vi "RT Driver VI.vi"(7 "Operation":T6, 11 "Device Reference in":T7 format="%.0x") -> (0 "Error Code":i32)   [LabVIEW 2027, in "Embedded Data Logger Engine.lvlib"]
uses:
  Embedded Data Logger Engine.lvlib
  <vilib>/NI VeriStand/Custom Device API/Custom Device Item Ref.ctl
  <vilib>/NI VeriStand/Custom Device API/Hardware Interface Driver VI Operation.ctl
  Embedded Data Logger State Data.ctl
  File Sampling Specification.ctl
  <vilib>/NI VeriStand/Custom Device API/Data Reference.ctl
  Group Sampling Specification.ctl
  <vilib>/NI VeriStand/Custom Device API/Block Data Reference.ctl
  <vilib>/NI VeriStand/Custom Device API/Get Item Property (I32).vi
  <vilib>/NI VeriStand/Custom Device API/Global Data Refs.vi
  <vilib>/NI VeriStand/Custom Device API/Custom Device API.lvlib
panel:
  in  "State":T1 {"FIFO % Ref" format="%.0x"; "Error Ref" format="%.0x"; "File Sample Specs"."File Status Ref" format="%.0x"; "File Sample Specs"."Cmd Ref" format="%.0x"; "File Sample Specs"."Data Loss Ref" format="%.0x"; "File Sample Specs"."Error Ref" format="%.0x"; "File Sample Specs"."Groups"."Decimation Ref" format="%.0x"; "File Sample Specs"."Groups"."Block Refs"."Data Reference" format="%.0x"; "File Sample Specs"."Trigger Ref" format="%.0x"}
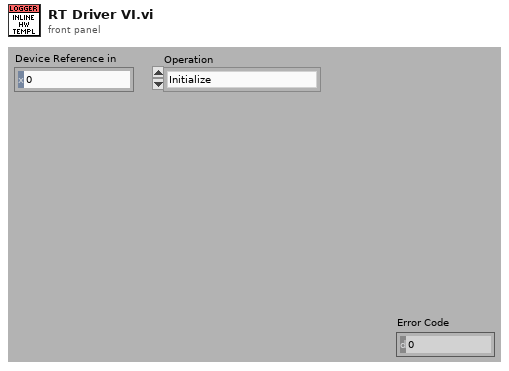
[diagram p1: front panel]
types:
  T1 = typedef "Embedded Data Logger Engine.lvlib/Embedded Data Logger State Data.ctl" = cluster{"File Sample Specs":T2[], "Data FIFO":refnum<k33>, "Data FIFO Buffer":dbl[], "error":errorcluster, "Stat FIFO":refnum<k33>, "Stat FIFO Buffer":dbl[], "Error Ref":T3, "Buffer %":dbl, "Used Buffer Size":u32, "FIFO % Ref":T3}
  T2 = typedef "Embedded Data Logger Engine.lvlib/File Sampling Specification.ctl" = cluster{"ID":dbl, "Trigger Ref":T3, "Error Ref":T3, "Groups":T4[], "Pretrigger":bool, "Data Loss Ref":T3, "Loss Count":i32, "Update Count":bool, "Cmd Ref":T3, "File Status Ref":T3, "Last Trigger Value":bool, "File requested to be open":bool}
  T3 = typedef "Custom Device API.lvlib/Data Reference.ctl" = i32
  T4 = typedef "Embedded Data Logger Engine.lvlib/Group Sampling Specification.ctl" = cluster{"ID":dbl, "Block Refs":T5[], "Data":dbl[], "Decimation":i32, "Counter":i32, "Decimation Ref":T3}
  T5 = typedef "Custom Device API.lvlib/Block Data Reference.ctl" = cluster{"Data Reference":T3, "Offset":u64, "Length":u64}
  T6 = typedef "Custom Device API.lvlib/Hardware Interface Driver VI Operation.ctl" = enum16{"Initialize", "Start", "Read Data from HW", "Write Data to HW", "Close"}
  T7 = typedef "Custom Device API.lvlib/Custom Device Item Ref.ctl" = u64
  T8 = cluster{"read mode":enum16{"polling", "blocking"}, "write mode":enum16{"polling", "blocking"}}
  T9 = typedef "Embedded Data Logger Engine.lvlib/File Logging Specification.ctl" = cluster{"Directory":path, "Groups":T10[], "Buffer Size":i32, "Properties":T12[], "Pretrigger":bool, "Pretrigger Samples":i32, "Name":string, "Timestamp":bool, "Error":i32, "Auto Open":bool, "File Node Ref":T7, "Archive":bool, "Archive Directory":path, "Segment Files":bool, "Segment Files By":T13, "Segment Size":u32, "Flushed Data Size Total":u32, "Append Waveform Properties":bool, "Logging State":T14, "First Sample Start Time":timestamp, "System dt":dbl}
  T10 = typedef "Embedded Data Logger Engine.lvlib/Group Logging Specification.ctl" = cluster{"Name":string, "Description":string, "Channels":string[], "Buffer Data":T11, "Channel Properties":cluster{"Properties":T12[]}[], "dt":dbl}
  T11 = typedef "Embedded Data Logger Engine.lvlib/Group Buffer Data.ctl" = cluster{"Last":i32, "Start":i32, "Length":i32, "Channel Count":i32, "Data":dbl[][], "Last Trigger":bool}
  T12 = typedef "Embedded Data Logger Engine.lvlib/Property Specification.ctl" = cluster{"Name":string, "Value":variant}
  T13 = typedef "Embedded Data Logger Shared.lvlib/Segment Files By.ctl" = enum16{"Time", "Size"}
  T14 = typedef "Embedded Data Logger Engine.lvlib/Logging State.ctl" = enum16{"Not Started", "Continous Logging", "Paused", "Discontinous Logging"}
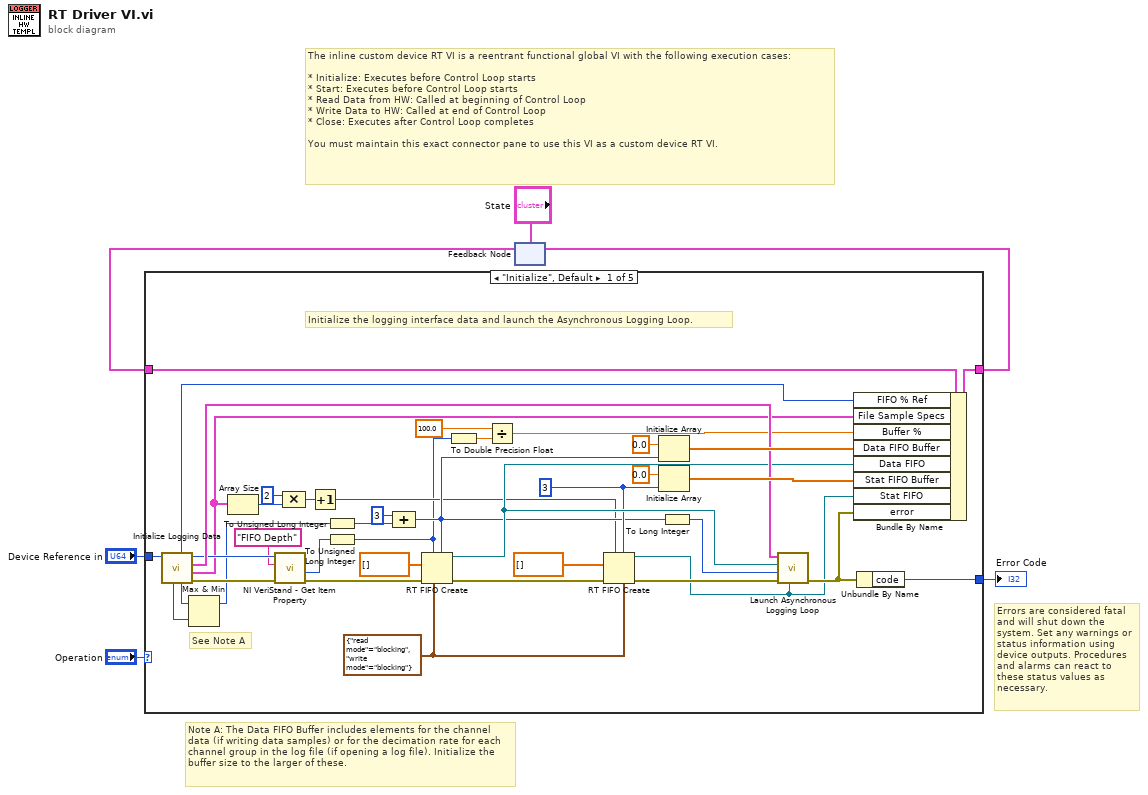
[diagram p0: block diagram]
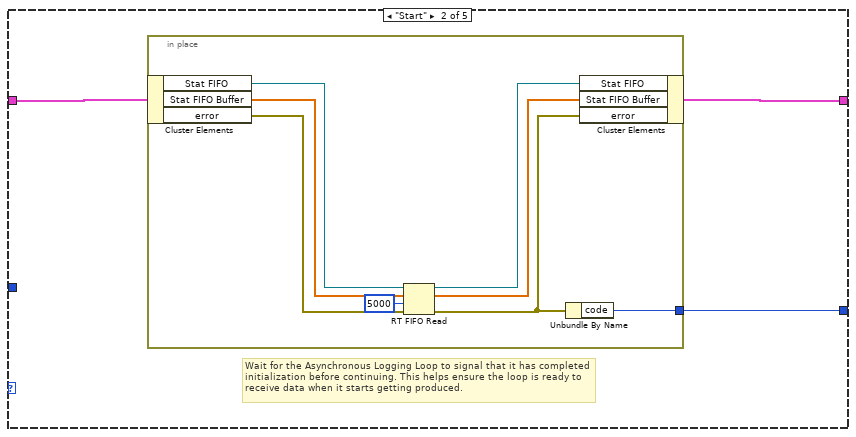
[diagram p2: hidden frame]
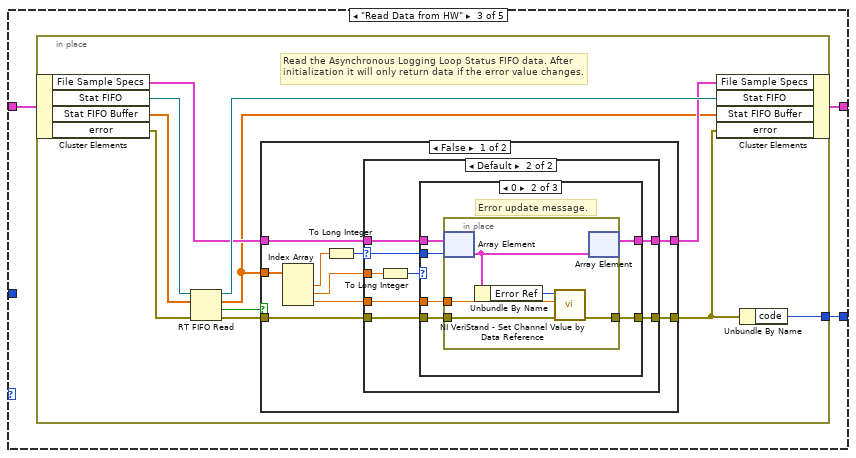
[diagram p3: hidden frame]
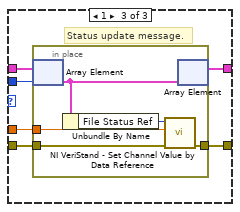
[diagram p6: hidden frame]
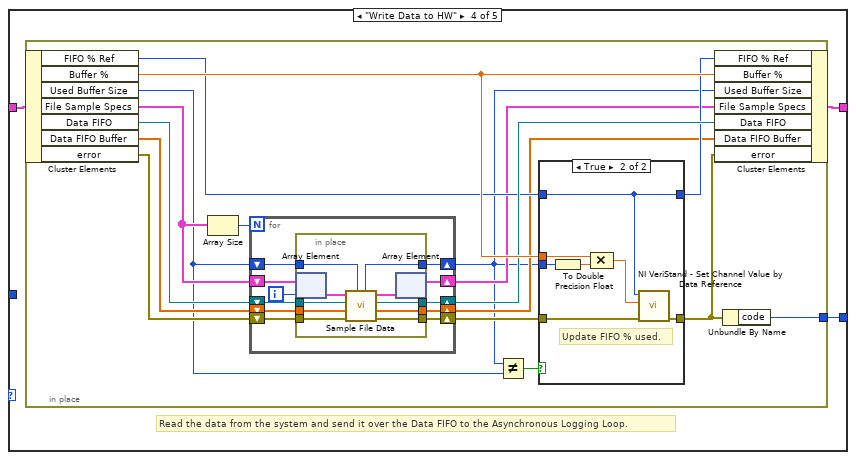
[diagram p8: hidden frame]
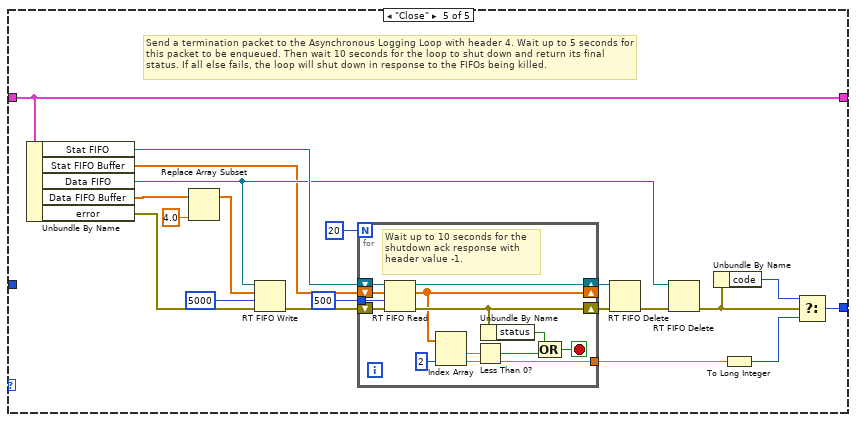
[diagram p10: hidden frame]
diagram:
  # "Note A: The Data FIFO Buffer includes elements for the channel data (if writing data samples) or for the decimation rate for each channel group in the log file (if opening a log file). Initialize the buffer size to the larger of these."
  # "Errors are considered fatal and will shut down the system. Set any warnings or status information using device outputs. Procedures and alarms can react to these status values as necessary."
  # "The inline custom device RT VI is a reentrant functional global VI with the following execution cases:\n\n* Initialize: Executes before Control Loop starts\n* Start: Executes before Control Loop starts\n* Read Data from HW: Called at beginning of Control Loop\n* Write Data to HW: Called at end of Control Loop\n* Close: Executes after Control Loop completes\n\nYou must maintain this exact connector pane to use this VI as a custom device RT VI."
  n1 = feedback #1("State") -> (w4:T1)
  n2 = case shown="\"Initialize\", Default" "Operation" {
    tunnel: "Device Reference in" -> [w41 _ _ _ _]
    tunnel: w4 -> [w17 w48 w59 w119 w182]
    tunnel: [w33 w49 w60 w117 w168] -> w3
    tunnel: [w16 w47 w58 w118 w182] -> w2
    frame "Initialize", Default {
      w28 = T8 {"read mode"=enum."blocking", "write mode"=enum."blocking"} ("r/w modes (polling,polling)")
      w29 = u32 3 ("elements in array (1)")
      # "See Note A"
      # "Initialize the logging interface data and launch the Asynchronous Logging Loop."
      n3 = call "Initialize Logging Data.vi"("Device Ref in"=w41) -> ("error out"=w38:errorcluster, "File Sample Specs"=w23:T2[], "File Log Specs"=w44:T9[], "Device Ref out"=w42:T7, "Max Group Size"=w8:i32, "FIFO % Ref"=w15:T3, "Max # Channel Groups"=w9:i32)  [unwired: 1 in, 3 out]
      n4 = Max & Min(x=w8, y=w9) -> (max(x,y)=w7:i32)  [unwired: 1 out]
      n5 = Array Size(array=w23) -> (size(s)=w22:i32)
      n6 = call-poly <vilib>:"NI VeriStand - Get Item Property.vi"("error in (no error)"=w38, "Property Name"="FIFO Depth", "Item Ref in"=w42) -> ("error out"=w37:errorcluster, "Value"=w19:i32)  [unwired: 1 in, 6 out]
      n7 = Compound Arithmetic op=MULTIPLY(2 ("value"), w22) -> (w11:i32)
      n8 = Increment(x=w11) -> (x+1=w21:i32)
      n9 = To Unsigned Long Integer(number=w7) -> (unsigned 32bit integer=w36:u32)
      n10 = To Unsigned Long Integer(number=w19) -> (unsigned 32bit integer=w18:u32)
      n11 = Compound Arithmetic op=ADD(u32 3 ("value"), w36) -> (w25:u32)
      n12 = RT FIFO Create(1:dbl[] [], 3:w37, 4:w18, 6:w25, 7:w28) -> (8:w43:refnum<k33>, 11:w31:errorcluster)  [unwired: 1 in, 3 out]
      n13 = To Double Precision Float(number=w18) -> (double precision float=w12:dbl)
      n14 = Divide(x=100.0, y=w12) -> (x/y=w14:dbl)
      n15 = RT FIFO Create(1:dbl[] [], 3:w31, 4:w21, 6:w29, 7:w28) -> (8:w24:refnum<k33>, 11:w27:errorcluster)  [unwired: 1 in, 3 out]
      n16 = Initialize Array(0.0 ("element"), w25) -> (w45:dbl[])
      n17 = Initialize Array(0.0 ("element"), w29) -> (w46:dbl[])
      n18 = To Long Integer(number=w25) -> (32bit integer=w20:i32)
      n19 = call "Launch Asynchronous Logging Loop.vi"("Log Status FIFO"=w24, "error in (no error)"=w27, "Log Data FIFO Size"=w20, "Log Data FIFO"=w43, "File Logging Specs"=w44) -> ("error out"=w26:errorcluster)  [unwired: 6 in]
      n20 = Bundle By Name(cluster=w17, "FIFO % Ref"=w15, "File Sample Specs"=w23, "Buffer %"=w14, "Data FIFO Buffer"=w45, "Data FIFO"=w43, "Stat FIFO Buffer"=w46, "Stat FIFO"=w24, "error"=w26) -> (w16:T1)
      n21 = Unbundle By Name(w26) -> ("code"=w33:i32)
    }
    frame "Start" {
      # "Wait for the Asynchronous Logging Loop to signal that it has completed initialization before continuing. This helps ensure the loop is ready to receive data when it starts getting produced."
      n22 = in-place {
        in-place-border: [w56] -> w49
        n23 = in-place-cluster #2(w48) -> ("Stat FIFO"=w55:refnum<k33>, "Stat FIFO Buffer"=w54:dbl[], "error"=w53:errorcluster)
        n24 = RT FIFO Read(0:w55, 1:w54, 2:5000 ("timeout in ms (0)"), 3:w53) -> (8:w52:refnum<k33>, 9:w51:dbl[], 11:w50:errorcluster)  [unwired: 2 out]
        n25 = Unbundle By Name(w50) -> ("code"=w56:i32)
        n26 = in-place-cluster #2("Stat FIFO"=w52, "Stat FIFO Buffer"=w51, "error"=w50) -> (w47:T1)
      }
    }
    frame "Read Data from HW" {
      n27 = in-place {
        in-place-border: [w67] -> w60
        # "Read the Asynchronous Logging Loop Status FIFO data. After initialization it will only return data if the error value changes."
        n28 = in-place-cluster #3(w59) -> ("File Sample Specs"=w66:T2[], "Stat FIFO"=w65:refnum<k33>, "Stat FIFO Buffer"=w64:dbl[], "error"=w63:errorcluster)
        n29 = RT FIFO Read(0:w65, 1:w64, 3:w63) -> (8:w71:refnum<k33>, 9:w62:dbl[], 10:w69:bool, 11:w68:errorcluster)  [unwired: 2 out]
        n30 = case shown="False" w69 {
          tunnel: w62 -> [w80 _]
          tunnel: w66 -> [w78 w115]
          tunnel: w68 -> [w77 w116]
          tunnel: [w76 w116] -> w61
          tunnel: [w74 w115] -> w70
          frame False {
            n31 = Index Array(array=w80) -> (element #1=w79:dbl, element #2=w72:dbl, element #3=w73:dbl)  [unwired: 3 in]
            n32 = To Long Integer(number=w79) -> (32bit integer=w75:i32)
            n33 = case shown="Default" w75 {
              selector: w75 -> [_ w86]
              tunnel: w78 -> [w81 w87]
              tunnel: w73 -> [_ w90]
              tunnel: w77 -> [w82 w89]
              tunnel: [w82 w88] -> w76
              tunnel: [w81 w85] -> w74
              tunnel: w72 -> [_ w84]
              frame -1 {
              }
              frame Default {
                n34 = To Long Integer(number=w84) -> (32bit integer=w83:i32)
                n35 = case shown="0" w83 {
                  tunnel: w90 -> [_ w98 w109]
                  tunnel: w89 -> [w91 w97 w108]
                  tunnel: [w91 w96 w107] -> w88
                  tunnel: w87 -> [w92 w95 w106]
                  tunnel: w86 -> [_ w94 w105]
                  tunnel: [w92 w93 w104] -> w85
                  frame Default {
                  }
                  frame 0 {
                    # "Error update message."
                    n36 = in-place {
                      in-place-border: w98 -> [w103]
                      in-place-border: w97 -> [w102]
                      in-place-border: [w101] -> w96
                      n37 = in-place-array #4(w95, w94) -> (w99:T2)
                      n38 = Unbundle By Name(w99) -> ("Error Ref"=w100:T3)
                      n39 = call <vilib>:"NI VeriStand - Set Channel Value by Data Reference.vi"("error in (no error)"=w102, "Value"=w103, "Data Reference in"=w100) -> ("error out"=w101:errorcluster)  [unwired: 8 out]
                      n40 = in-place-array #4(w99) -> (w93:T2[])  [unwired: 1 out]
                    }
                  }
                  frame 1 {
                    # "Status update message."
                    n41 = in-place {
                      in-place-border: w109 -> [w114]
                      in-place-border: w108 -> [w113]
                      in-place-border: [w112] -> w107
                      n42 = in-place-array #5(w106, w105) -> (w110:T2)
                      n43 = Unbundle By Name(w110) -> ("File Status Ref"=w111:T3)
                      n44 = call <vilib>:"NI VeriStand - Set Channel Value by Data Reference.vi"("error in (no error)"=w113, "Value"=w114, "Data Reference in"=w111) -> ("error out"=w112:errorcluster)  [unwired: 8 out]
                      n45 = in-place-array #5(w110) -> (w104:T2[])  [unwired: 1 out]
                    }
                  }
                }
              }
            }
          }
          frame True {
            # "No error value reported."
          }
        }
        n46 = in-place-cluster #3("File Sample Specs"=w70, "Stat FIFO"=w71, "Stat FIFO Buffer"=w62, "error"=w61) -> (w58:T1)
        n47 = Unbundle By Name(w61) -> ("code"=w67:i32)
      }
    }
    frame "Write Data to HW" {
      # "Read the data from the system and send it over the Data FIFO to the Asynchronous Logging Loop."
      n48 = in-place {
        in-place-border: [w130] -> w117
        n49 = in-place-cluster #6(w119) -> ("FIFO % Ref"=w124:T3, "Buffer %"=w136:dbl, "Used Buffer Size"=w129:u32, "File Sample Specs"=w135:T2[], "Data FIFO"=w133:refnum<k33>, "Data FIFO Buffer"=w132:dbl[], "error"=w131:errorcluster)
        n50 = Array Size(array=w135) -> (size(s)=w134:i32)
        n51 = for {
          N: w134 -> [_]
          shift-right: [w155] -> w122
          shift-left: w135 -> [w156]
          shift-right: [w152] -> w128
          shift-left: w133 -> [w153]
          shift-right: [w150] -> w121
          shift-left: w132 -> [w151]
          shift-right: [w148] -> w126
          shift-left: w131 -> [w149]
          shift-right: [w146] -> w120
          shift-left: w129 -> [w147]
          i -> [w154]
          n52 = in-place {
            in-place-border: w153 -> [w164]
            in-place-border: [w163] -> w152
            in-place-border: w151 -> [w162]
            in-place-border: [w161] -> w150
            in-place-border: w149 -> [w160]
            in-place-border: [w159] -> w148
            in-place-border: w147 -> [w158]
            in-place-border: [w157] -> w146
            n53 = in-place-array #7(w156, w154) -> (w166:T2)
            n54 = call "Sample File Data.vi"("Buffer Used in"=w158, "error in (no error)"=w160, "Data FIFO Buffer in"=w162, "Data FIFO in"=w164, "File Sample Spec in"=w166) -> ("error out"=w159:errorcluster, "Data FIFO Buffer out"=w161:dbl[], "Data FIFO out"=w163:refnum<k33>, "File Sample Spec out"=w165:T2, "Buffer Used out"=w157:u32)  [unwired: 2 out]
            n55 = in-place-array #7(w165) -> (w155:T2[])  [unwired: 1 out]
          }
        }
        n56 = Not Equal?(x=w120, y=w129) -> (x != y?=w127:bool)
        n57 = case shown="True" w127 {
          tunnel: w126 -> [w138 w145]
          tunnel: [w138 w144] -> w125
          tunnel: w124 -> [w137 w143]
          tunnel: [w137 w143] -> w123
          tunnel: w120 -> [_ w142]
          tunnel: w136 -> [_ w139]
          frame False {
          }
          frame True {
            # "Update FIFO % used."
            n58 = To Double Precision Float(number=w142) -> (double precision float=w141:dbl)
            n59 = Compound Arithmetic op=MULTIPLY(w139, w141) -> (w140:dbl)
            n60 = call <vilib>:"NI VeriStand - Set Channel Value by Data Reference.vi"("error in (no error)"=w145, "Value"=w140, "Data Reference in"=w143) -> ("error out"=w144:errorcluster)  [unwired: 8 in]
          }
        }
        n61 = in-place-cluster #6("FIFO % Ref"=w123, "Buffer %"=w136, "Used Buffer Size"=w120, "File Sample Specs"=w122, "Data FIFO"=w128, "Data FIFO Buffer"=w121, "error"=w125) -> (w118:T1)
        n62 = Unbundle By Name(w125) -> ("code"=w130:i32)
      }
    }
    frame "Close" {
      # "Send a termination packet to the Asynchronous Logging Loop with header 4. Wait up to 5 seconds for this packet to be enqueued. Then wait 10 seconds for the loop to shut down and return its final status. If all else fails, the loop will shut down in response to the FIFOs being killed."
      n63 = Unbundle By Name(w182) -> ("Stat FIFO"=w186:refnum<k33>, "Stat FIFO Buffer"=w176:dbl[], "Data FIFO"=w184:refnum<k33>, "Data FIFO Buffer"=w180:dbl[], "error"=w181:errorcluster)
      n64 = Replace Array Subset(array=w180, new element=4.0 ("new element/subarray")) -> (w178:dbl[])  [unwired: 1 in]
      n65 = RT FIFO Write(0:w184, 1:w178, 2:5000 ("timeout in ms (0)"), 3:w181) -> (11:w172:errorcluster)  [unwired: 1 in, 3 out]
      n66 = for {
        N: 20 -> [_]
        tunnel: [w193] -> w175
        tunnel: 500 ("timeout in ms (0)") -> [w195]
        shift-right: [w197] -> w183
        shift-left: w186 -> [w198]
        shift-right: [w199] -> w185
        shift-left: w172 -> [w194]
        shift-right: [w187] -> _
        shift-left: w176 -> [w196]
        stop <- w189 stop-if-true
        # "Wait up to 10 seconds for the shutdown ack response with header value -1."
        n67 = RT FIFO Read(0:w198, 1:w196, 2:w195, 3:w194) -> (8:w197:refnum<k33>, 9:w187:dbl[], 11:w199:errorcluster)  [unwired: 2 out]
        n68 = Index Array(array=w187, index #2=2 ("index")) -> (element #1=w191:dbl, element #2=w193:dbl)  [unwired: 1 in]
        n69 = Less Than 0?(x=w191) -> (x < 0?=w190:bool)
        n70 = Unbundle By Name(w199) -> ("status"=w188:bool)
        n71 = Compound Arithmetic op=OR(w188, w190) -> (w189:bool)
      }
      n72 = RT FIFO Delete(0:w183, 3:w185) -> (11:w173:errorcluster)  [unwired: 1 in]
      n73 = RT FIFO Delete(0:w184, 3:w173) -> (11:w171:errorcluster)  [unwired: 1 in]
      n74 = Unbundle By Name(w171) -> ("code"=w170:i32)
      n75 = To Long Integer(number=w175) -> (32bit integer=w169:i32)
      n76 = Select(t=w170, s=w171, f=w169) -> (s? t:f=w168:i32)
    }
  }
  "Error Code" <- w3
  n77 = feedback-in #1(w2) -> ()
